vi "stopCallBack.vi"(8 "error in (no error)":errorcluster, 11 "TcpServerBase in":refnum<class "TcpServerBase.lvclass">) -> (0 "error out":errorcluster, 3 "TcpServerBase out":refnum<class "TcpServerBase.lvclass">)   [LabVIEW 2018, in "TcpServerBase.lvclass"]
doc: "Send a signal to stop the Sender Loop (inside of readWritePacket.vi)"
uses:
  TcpServerBase.lvclass
  TcpServerBase.lvclass/TcpServerBase.ctl
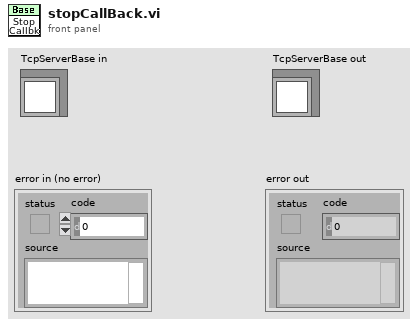
[diagram p1: front panel]
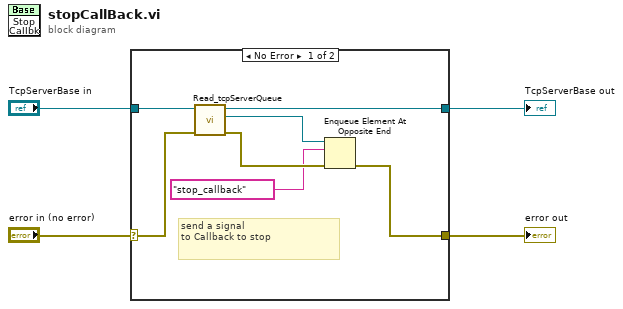
[diagram p0: block diagram]
diagram:
  n1 = case shown="No Error" "error in (no error)" {
    selector: "error in (no error)" -> [w7 w13]
    tunnel: [w6 w13] -> w3
    tunnel: [w9 w12] -> w1
    tunnel: "TcpServerBase in" -> [w10 w12]
    frame No Error {
      # "send a signal \nto Callback to stop"
      n2 = call "Read_tcpServerQueue.vi"("error in (no error)"=w7, "TcpServerBase in"=w10) -> ("error out"=w8:errorcluster, "tcpServerQueue"=w11:refnum<queue>, "TcpServerBase out"=w9:refnum<class "TcpServerBase.lvclass">)  [unwired: 7 in]
      n3 = Enqueue Element At Opposite End(queue=w11, element="stop_callback", error in (no error)=w8) -> (error out=w6:errorcluster)  [unwired: 1 in, 2 out]
    }
    frame Error {
    }
  }
  "error out" <- w3
  "TcpServerBase out" <- w1
